vi "Read RTD Temperature.vi"(11 "error in (no error)":errorcluster) -> (6 "Temperature (DegC)":dbl, 15 "error out":errorcluster)   [LabVIEW 2010]
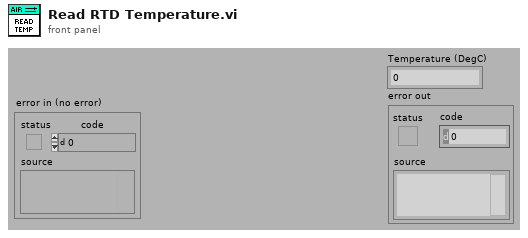
[diagram p1: front panel]
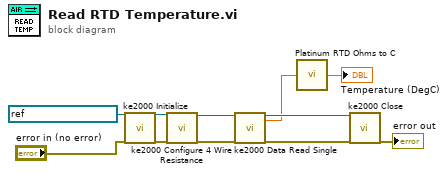
[diagram p0: block diagram]
diagram:
  n1 = call "ke2000 Initialize.vi"("VISA resource name"=refnum<visa-resource-name> "GPIB0::8::INSTR", "error in (no error)"="error in (no error)") -> ("VISA resource name out"=w10:refnum<visa-resource-name>, "error out"=w11:errorcluster)  [unwired: 16 in]
  n2 = call "ke2000 Configure 4 Wire Resistance.vi"("VISA resource name"=w10, "error in (no error)"=w11) -> ("VISA resource name out"=w6:refnum<visa-resource-name>, "error out"=w8:errorcluster)  [unwired: 16 in]
  n3 = call "ke2000 Data Read Single.vi"("VISA resource name"=w6, "error in (no error)"=w8) -> ("VISA resource name out"=w5:refnum<visa-resource-name>, "Measurement"=w2:dbl, "error out"=w7:errorcluster)  [unwired: 13 in, 2 out]
  n4 = call "Platinum RTD Ohms to C.vi"("Rt"=w2) -> ("Temp (C)"=→"Temperature (DegC)":dbl)
  n5 = call "ke2000 Close.vi"("VISA resource name"=w5, "error in (no error)"=w7) -> ("error out"=→"error out":errorcluster)  [unwired: 17 in]
